vi "Write Initial Data from String.vi"(1 "Data":string) -> (0 "Write OK":bool)   [LabVIEW 2012]
doc: "The Basic Serial Read and Write example performs a Serial Port Read, a Serial Port Write, or a combination of these actions. The user selects the actions (read or write) on the front panel. If both are selected, the VI will write the data first, read data, and then close the VISA session that is opened to the port. This VI will wait until the specified number of bytes is received at the port or until a termination character is read.\n\nINSTRUCTIONS:\n1) Select the serial resource and configuration parameters (baud rate, data bits, parity, stop bits, flow control).\n2) Select the operations to be performed. \n3) Connect the serial port to your device. If no device is available, perform a loopback test by doing one of the following. Short pins 2 and 3 on a RS-232 cable or short pin 4 to pin 8 and pin 5 to pin 9 on a RS-485/422 cable. \n4) Run the VI to see the data read. (The \"read string\" will match the \"string to write\" if a loopback test was performed.)\n\nNote: The parameters set for the serial port must match the parameters of the connected instrument or device. In this example, the bytes to read parameter specifies the number of bytes that the serial port reads. If there were more bytes at the port than the number specified in bytes to read, those bytes would not be read. Also, if you specify to read more bytes than the number of bytes actually read, you might receive a timeout error message.\n\nOn the block diagram, the Configure Serial Port VI sets the configuration parameters. The front panel displays the controls used to configure the basic parameters, such as baud rate, data bits, and parity. Constants configure the other parameters the user probably does not need set. After the VISA Configure Serial Port VI opens the VISA session and configures the port, the VI passes the VISA resource name to other VIs that perform operations on that VISA resource. The VISA Write function sends a command to the serial device and the VISA Read function returns data based on the command. The VISA Close function then closes the reference to the serial device. It is important to close the reference; otherwise communication through with that port through protocols other than VISA might not be possible."
uses:
  Correlator port.vi
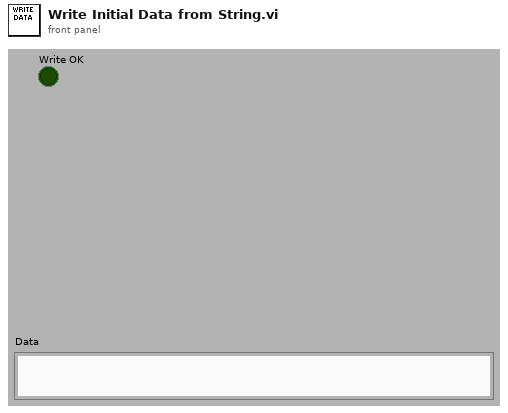
[diagram p1: front panel]
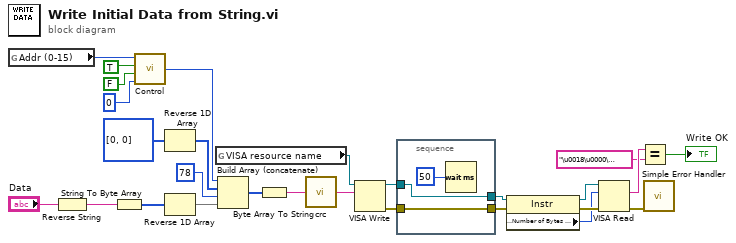
[diagram p0: block diagram]
diagram:
  n1 = global read "Correlator port.vi" "Addr (0-15)"() -> (w5:i8)
  n2 = Reverse String(1:"Data") -> (0:w7:string)
  n3 = String To Byte Array(string=w7) -> (unsigned byte array=w12:u8[])
  n4 = call "Control.vi"("Page"=i8 0, "Error"=FALSE, "Write"=TRUE, "Addr"=w5) -> ("Control Byte"=w17:u32)
  n5 = Reverse 1D Array(array=i8[] [0, 0] ("Offset")) -> (reversed array=w15:i8[])
  n6 = Reverse 1D Array(array=w12) -> (reversed array=w11:u8[])
  n7 = global read "Correlator port.vi" "VISA resource name"() -> (w6:refnum<visa-resource-name>)
  n8 = Build Array (concatenate)(w17, w15, u8 78 ("Length"), w11) -> (w10:u32[])
  n9 = Byte Array To String(unsigned byte array=w10) -> (string=w9:string)
  n10 = call "crc.vi"("Input string"=w9) -> ("Output (with crc)"=w8:string)
  n11 = VISA Write(VISA resource name=w6, write buffer=w8) -> (VISA resource name out=w25:refnum<visa-resource-name>, error out=w27:errorcluster)  [unwired: 1 in, 1 out]
  n12 = stacked-sequence {
    tunnel: w27 -> [w30]
    tunnel: [w30] -> w26
    tunnel: w25 -> [w29]
    tunnel: [w29] -> w24
    frame #0 {
      n13 = Wait (ms)(milliseconds to wait=u32 50 ("delay before read (ms)")) -> ()  [unwired: 1 out]
    }
  }
  n14 = property class="Instr"(reference=w24, error in=w26) -> (reference out=w4:refnum<visa-resource-name>, error out=w3:errorcluster, "Serial Settings:Number of Bytes at Serial Port"=w2:u32)
  n15 = VISA Read(VISA resource name=w4, byte count=w2, error in (no error)=w3) -> (read buffer=w23:string, error out=w1:errorcluster)  [unwired: 2 out]
  n16 = Equal?(x=w23, y="\u0018\u0000\u0000N:") -> (x = y?=→"Write OK":bool)
  n17 = call <vilib>:"Simple Error Handler.vi"("error in (no error)"=w1) -> ()  [unwired: 1 in, 8 out]
